vi "update_position.vi"(1 "Car.lvclass":refnum<class "Car.lvclass">, 2 "Obstacles":dbl[][](array[numeric]), 3 "Sonar Readngs (mm)":dbl[](array[numeric]), 4 "Time Since Last Update":dbl) -> (0 "Car.lvclass 2":refnum<class "Car.lvclass">)   [LabVIEW 2015]
uses:
  class/Car.lvclass
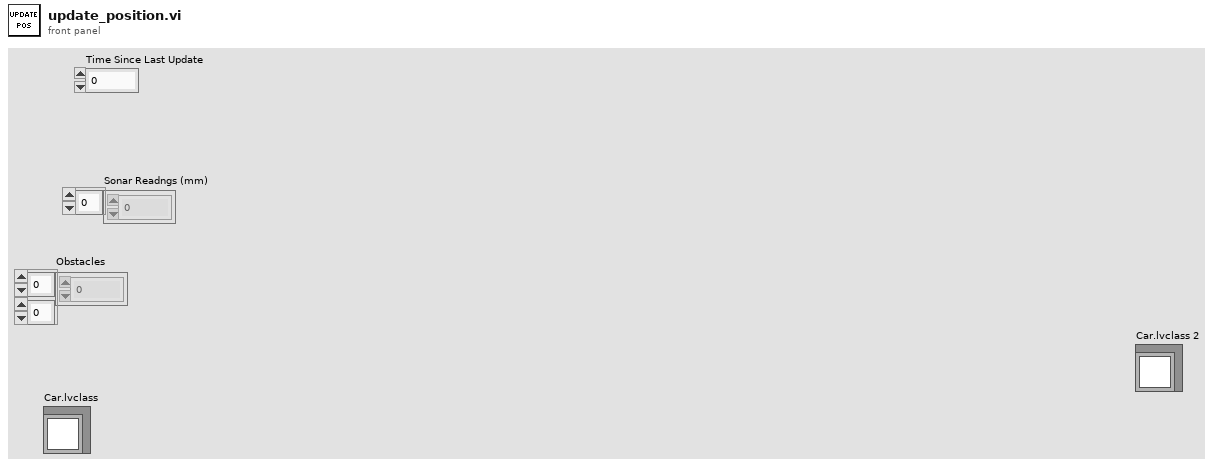
[diagram p1: front panel]
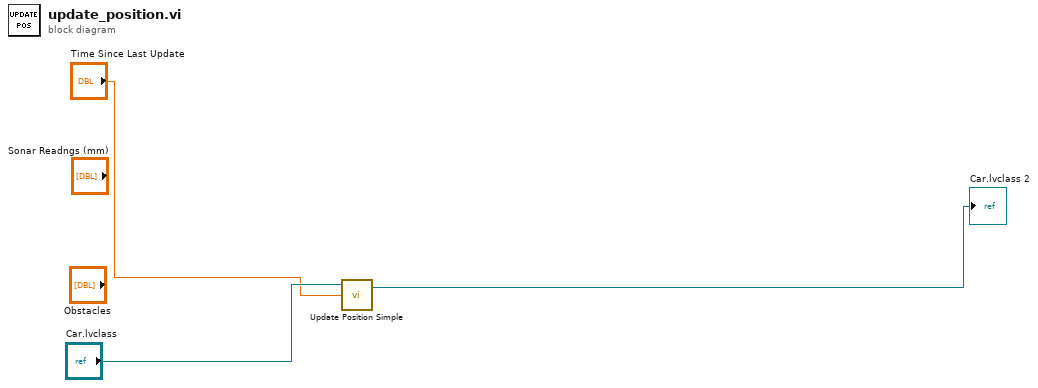
[diagram p0: block diagram]
diagram:
  n1 = call "Update Position Simple.vi"("Time Since Last Update"="Time Since Last Update", "Car.lvclass"="Car.lvclass") -> ("Car.lvclass 2"=→"Car.lvclass 2":refnum<class "Car.lvclass">)  [unwired: 1 in, 1 out]
